vi "addToLocalQ.vi"(8 "error in (no error)":errorcluster, 10 "ImageData":T1, 11 "CameraNetworkServer in":refnum<class "CameraNetworkServer.lvclass">) -> (0 "error out":errorcluster, 3 "CameraNetworkServer out":refnum<class "CameraNetworkServer.lvclass">)   [LabVIEW 2009, in "Hardware.lvlib" / "HWControllers.lvlib" / "CameraNetworkServer.lvclass"]
uses:
  CameraNetworkServer.lvclass
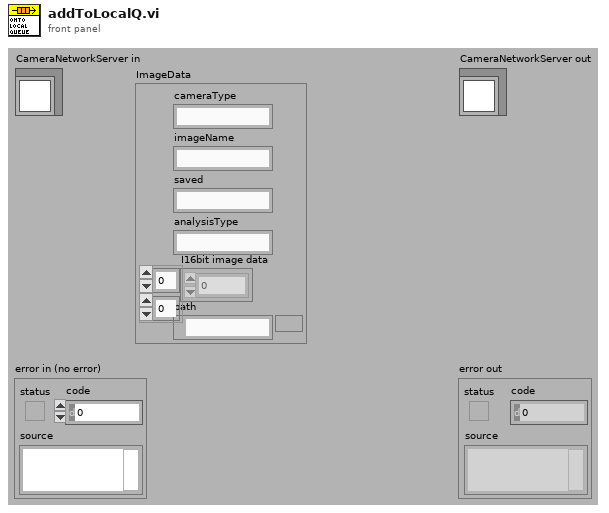
[diagram p1: front panel]
types:
  T1 = cluster{"cameraType":string, "imageName":string, "saved":string, "analysisType":string, "I16bit image data":i16[][], "path":path}
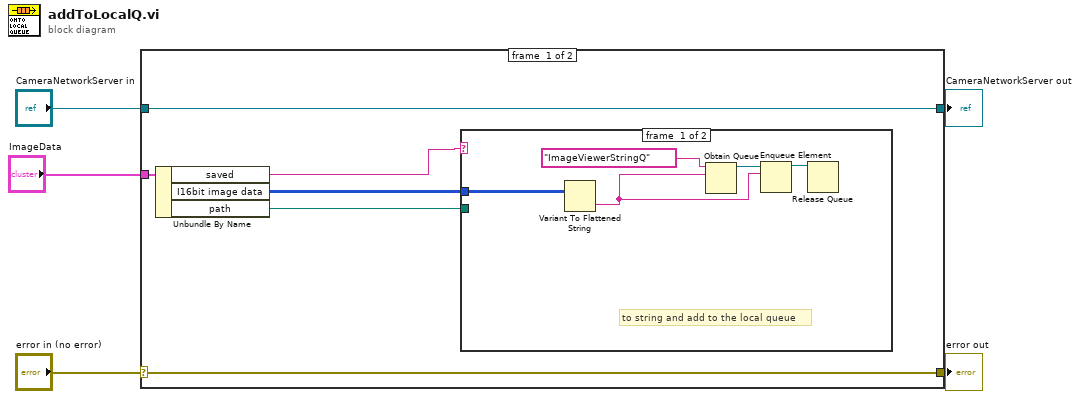
[diagram p0: block diagram]
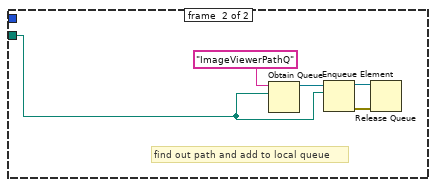
[diagram p2: hidden frame]
diagram:
  n1 = case shown="No Error" "error in (no error)" {
    selector: "error in (no error)" -> [w6 w23]
    tunnel: [w6 w23] -> w4
    tunnel: [w11 w22] -> w2
    tunnel: "CameraNetworkServer in" -> [w11 w22]
    tunnel: "ImageData" -> [w10 _]
    frame #0 {
      n2 = Unbundle By Name(w10) -> ("saved"=w9:string, "I16bit image data"=w8:i16[][], "path"=w7:path)
      n3 = case shown="\"false\", Default" w9 {
        tunnel: w8 -> [w12 _]
        tunnel: w7 -> [_ w17]
        frame #0 {
          # "to string and add to the local queue"
          n4 = Variant To Flattened String(Variant=w12) -> (data string=w13:string)  [unwired: 1 out]
          n5 = Obtain Queue(name (unnamed)="ImageViewerStringQ", element data type=w13) -> (queue out=w16:refnum<queue>)  [unwired: 3 in, 2 out]
          n6 = Enqueue Element(queue=w16, element=w13) -> (queue out=w15:refnum<queue>)  [unwired: 2 in, 2 out]
          n7 = Release Queue(queue=w15) -> ()  [unwired: 2 in, 3 out]
        }
        frame #1 {
          # "find out path and add to local queue"
          n8 = Obtain Queue(name (unnamed)="ImageViewerPathQ", element data type=w17) -> (queue out=w20:refnum<queue>)  [unwired: 3 in, 2 out]
          n9 = Enqueue Element(queue=w20, element=w17) -> (queue out=w19:refnum<queue>, error out=w18:errorcluster)  [unwired: 2 in, 1 out]
          n10 = Release Queue(queue=w19, error in (no error)=w18) -> ()  [unwired: 1 in, 3 out]
        }
      }
    }
    frame #1 {
    }
  }
  "error out" <- w4
  "CameraNetworkServer out" <- w2
